vi "makeScript.vi"(8 "error in (no error)":errorcluster caption="entrée d'erreur (pas d'erreur)", 10 "import":string, 11 "Model en entrée":refnum<class "Model.lvclass">) -> (0 "error out":errorcluster caption="sortie d'erreur", 3 "Model en sortie":refnum<class "Model.lvclass">)   [LabVIEW 2020, in "Model.lvclass"]
uses:
  Model.lvclass
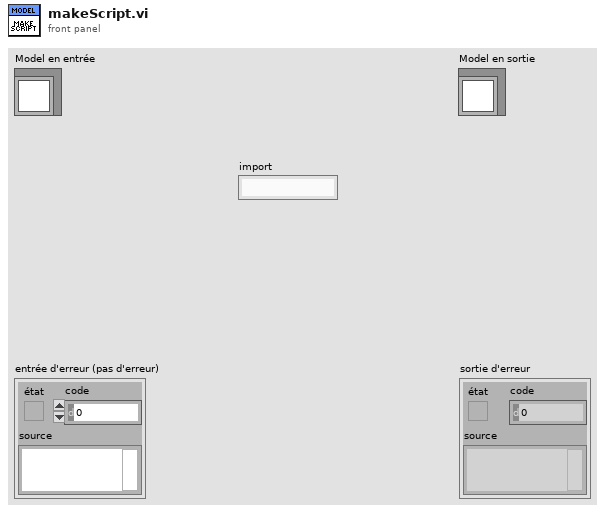
[diagram p1: front panel]
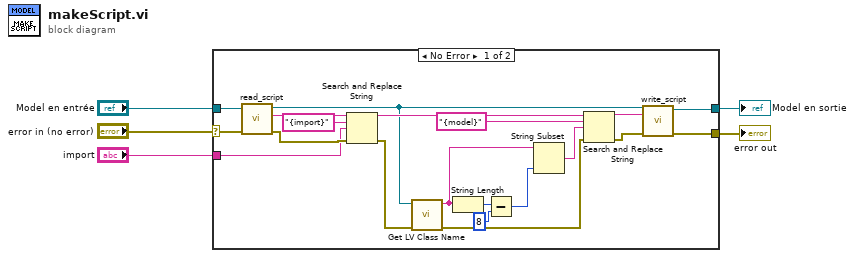
[diagram p0: block diagram]
diagram:
  n1 = case shown="No Error" "error in (no error)" {
    selector: "error in (no error)" -> [w7 w27]
    tunnel: [w6 w27] -> w4
    tunnel: [w8 w26] -> w2
    tunnel: "Model en entrée" -> [w25 w26]
    tunnel: "import" -> [w21 _]
    frame No Error {
      n2 = call-dynamic "read_script.vi"("error in (no error)"=w7, "Model en entrée"=w25) -> ("error out"=w22:errorcluster, "script"=w24:string, "Model en sortie"=w18:refnum<class "Model.lvclass">)  [unwired: 7 in]
      n3 = Search and Replace String(input string=w24, search string="{import}" ("chaîne recherchée"), replace string=w21, error in=w22) -> (result string=w20:string, error out=w17:errorcluster)  [unwired: 4 in, 2 out]
      n4 = call <vilib>:"Get LV Class Name.vi"("error in (no error)"=w17, "object"=w18) -> ("error out"=w10:errorcluster, "class name"=w14:string)  [unwired: 8 in]
      n5 = String Length(string=w14) -> (length=w16:i32)
      n6 = Subtract(x=w16, y=8) -> (x-y=w13:i32)
      n7 = String Subset(string=w14, length (rest)=w13) -> (substring=w12:string)  [unwired: 1 in]
      n8 = Search and Replace String(input string=w20, search string="{model}" ("chaîne recherchée"), replace string=w12, error in=w10) -> (result string=w11:string, error out=w9:errorcluster)  [unwired: 4 in, 2 out]
      n9 = call-dynamic "write_script.vi"("error in (no error)"=w9, "script"=w11, "Model en entrée"=w18) -> ("error out"=w6:errorcluster, "Model en sortie"=w8:refnum<class "Model.lvclass">)  [unwired: 7 in]
    }
    frame Error {
    }
  }
  "error out" <- w4
  "Model en sortie" <- w2
